vi "CheckSignal.vi"(8 "error in (no error)":errorcluster, 10 "Signals Specs Info":T1[](array[typedef]), 11 "Signals":i16[][](array[numeric])) -> (0 "error out":errorcluster, 2 "Init vals correct":bool[](array[boolean]), 3 "Checksums correct":bool[](array[boolean]))   [LabVIEW 2012]
doc: "Checks if a Physionet record is valid according to checksums and initial values read from header file."
uses:
  #TD_SignalSpecInfo.ctl
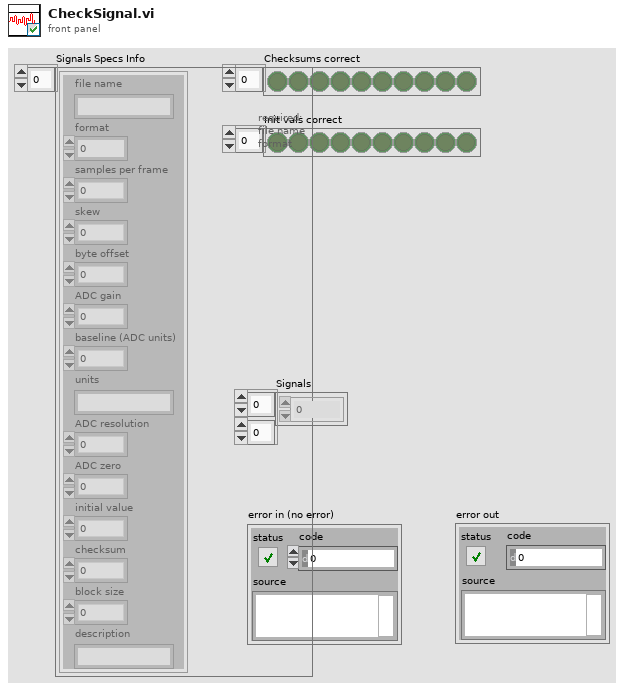
[diagram p1: front panel]
types:
  T1 = typedef "#TD_SignalSpecInfo.ctl" = cluster{"file name":string, "format":i32, "samples per frame":i32, "skew":i32, "byte offset":i32, "ADC gain":dbl, "baseline (ADC units)":i16, "units":string, "ADC resolution":i16, "ADC zero":i16, "initial value":i16, "checksum":i16, "block size":i32, "description":string}
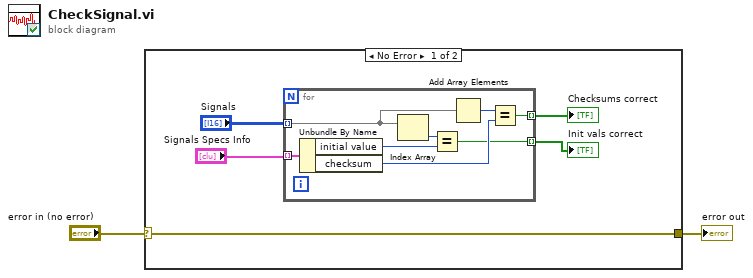
[diagram p0: block diagram]
diagram:
  n1 = case shown="No Error" "error in (no error)" {
    selector: "error in (no error)" -> [w3 w16]
    tunnel: [w3 w16] -> w1
    frame No Error {
      n2 = for {
        tunnel: "Signals" -> [w10] mode=indexing
        tunnel: "Signals Specs Info" -> [w11] mode=indexing
        tunnel: [w9] -> w6 mode=indexing
        tunnel: [w8] -> w7 mode=indexing
        n3 = Unbundle By Name(w11) -> ("initial value"=w15:i16, "checksum"=w13:i16)
        n4 = Index Array(array=w10) -> (element=w14:i16)  [unwired: 1 in]
        n5 = Equal?(x=w14, y=w15) -> (x = y?=w8:bool)
        n6 = Add Array Elements(numeric array=w10) -> (sum=w12:i16)
        n7 = Equal?(x=w12, y=w13) -> (x = y?=w9:bool)
      }
      "Checksums correct" <- w6
      "Init vals correct" <- w7
    }
    frame Error {
    }
  }
  "error out" <- w1
